vi "FTW-Actor-CheckShutdown.vi"(0 "FTW Actor Instance":refnum<class "FTW-ActorInstance.lvclass">, 11 "error in":errorcluster) -> (4 "FTW Actor Instance out":refnum<class "FTW-ActorInstance.lvclass">, 6 "Shutdown?":bool, 15 "error out":errorcluster)   [LabVIEW 2012, in "FTW-Actor.lvlib" / "FTW-ActorInstance.lvclass"]
uses:
  FTW-ActorInstance.lvclass
  FTW-ActorInstance.lvclass/FTW-ActorInstance.ctl
  JobSequencer/FTW-JobSequencer.lvclass/FTW-JobSequencer.ctl
  JobSequencer/FTW-JobSequencer.lvclass
panel:
  # "Inputs"
  # "Outputs"
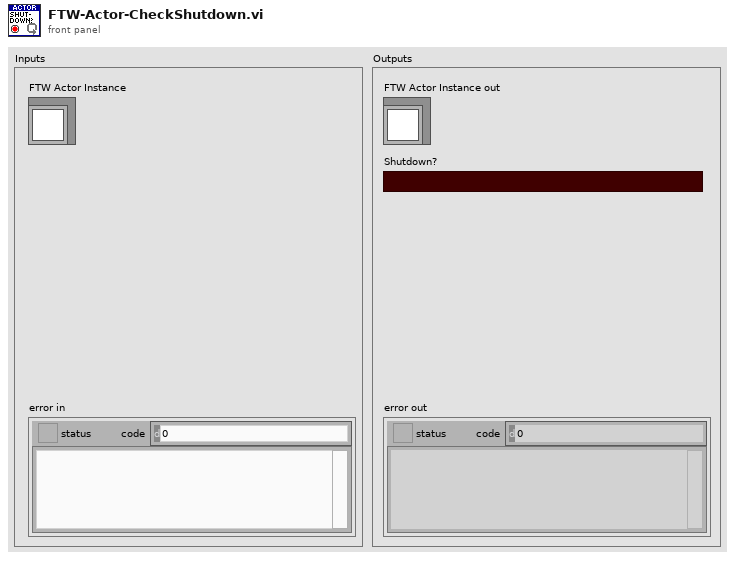
[diagram p1: front panel]
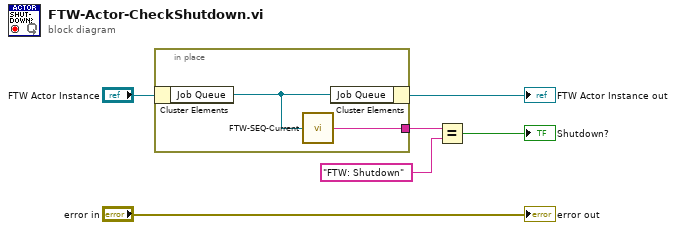
[diagram p0: block diagram]
diagram:
  n1 = in-place {
    in-place-border: [w8] -> w5
    n2 = in-place-cluster #1("FTW Actor Instance") -> ("Job Queue"=w7:refnum<class "FTW-JobSequencer.lvclass">)
    n3 = call "FTW-SEQ-Current.vi"("FTW Job Sequencer"=w7) -> ("Current Job"=w8:string)
    n4 = in-place-cluster #1("Job Queue"=w7) -> (→"FTW Actor Instance out":refnum<class "FTW-ActorInstance.lvclass">)
  }
  n5 = Equal?(x=w5, y="FTW: Shutdown") -> (x = y?=→"Shutdown?":bool)
  "error out" <- "error in"
